vi "Send Message.vi"(8 "error in (no error)":errorcluster, 10 "Message":string, 11 "Chat Client in":refnum<class "Chat Client.lvclass">) -> (0 "error out":errorcluster, 3 "Chat Client out":refnum<class "Chat Client.lvclass">)   [LabVIEW 2020, in "Chat Client.lvclass"]
uses:
  Chat Client.lvclass
  Chat Client.lvclass/Chat Client.ctl
  Stream-TCP/TCP Client/TCP Client.lvclass
  lv-stream/stream/Stream/Stream.lvclass
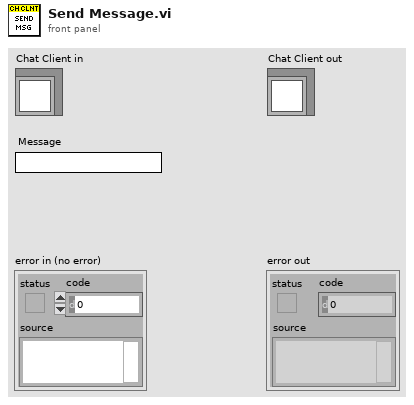
[diagram p1: front panel]
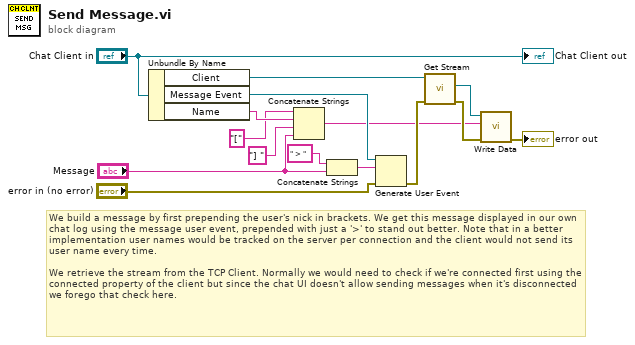
[diagram p0: block diagram]
diagram:
  # "We build a message by first prepending the user's nick in brackets. We get this message displayed in our own chat log using the message user event, prepended with just a '>' to stand out better. Note that in a better implementation user names would be tracked on the server per connection and the client would not send its user name every time.\n\nWe retrieve the stream from the TCP Client. Normally we would need to check if we're connected first using the connected property of the client but since the chat UI doesn't allow sending messages when it's disconnected we forego that check here."
  n1 = Unbundle By Name("Chat Client in") -> ("Client"=w7:refnum<class "TCP Client.lvclass">, "Message Event"=w9:refnum<user-event>, "Name"=w14:string)
  n2 = Concatenate Strings("[" ("string"), w14, "] " ("string"), "Message") -> (w2:string)
  n3 = Concatenate Strings(" > " ("string"), "Message") -> (w8:string)
  n4 = Generate User Event(user event=w9, event data cluster=w8, error in="error in (no error)") -> (error out=w5:errorcluster)  [unwired: 1 in, 1 out]
  n5 = call-dynamic "Get Stream.vi"("error in (no error)"=w5, "TCP Client in"=w7) -> ("error out"=w3:errorcluster, "Stream"=w4:refnum<class "Stream.lvclass">)  [unwired: 7 in, 1 out]
  n6 = call-dynamic "Write Data.vi"("error in (no error)"=w3, "Data"=w2, "Stream in"=w4) -> ("error out"=→"error out":errorcluster)  [unwired: 7 in, 1 out]
  "Chat Client out" <- "Chat Client in"
